vi "test_output_gain.vi"() -> ()   [LabVIEW 2025]
uses:
  test_x410/FPGA/IQ-1element.ctl
  <instrlib>/_niInstr/DSP/v1/Shared/Public/IQ Data.ctl
  <instrlib>/_niInstr/DSP/v1/Shared/niInstr DSP v1 Shared.lvlib
panel:
  in  "gain":fxp<+/-,16,10>
  in  "data in":T1=[{"I"=0.0, "Q"=0.0, "overflow"=FALSE}]
  out "I":fxp<+/-,18,1>
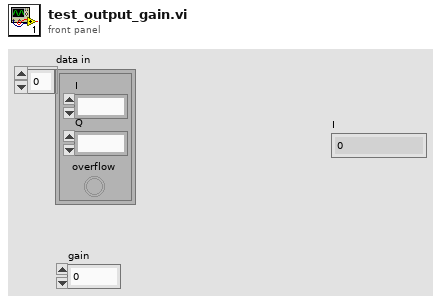
[diagram p1: front panel]
types:
  T1 = typedef "IQ-1element.ctl" = T2[]
  T2 = typedef "niInstr DSP v1 Shared.lvlib/IQ Data.ctl" = cluster{"I":fxp<+/-,18,1>, "Q":fxp<+/-,18,1>, "overflow":bool}
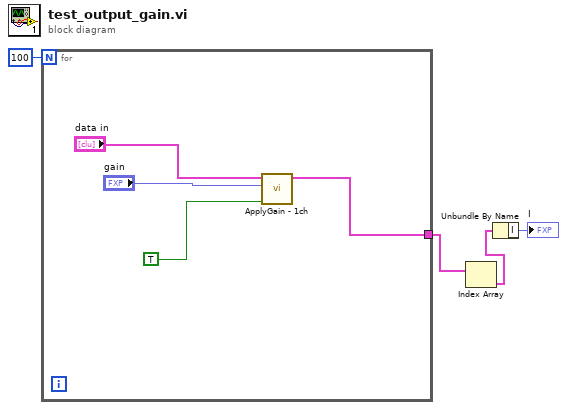
[diagram p0: block diagram]
diagram:
  n1 = for {
    N: 100 -> [_]
    tunnel: [w5] -> w3
    n2 = call "ApplyGain - 1ch.vi"("input valid"=TRUE ("valid in"), "gain"="gain", "data in"="data in") -> ("data out"=w5:T2[])  [unwired: 7 in, 1 out]
  }
  n3 = Index Array(array=w3) -> (element=w2:T2)  [unwired: 1 in]
  n4 = Unbundle By Name(w2) -> ("I"=→"I":fxp<+/-,18,1>)
